vi "Get Calibration Settings.vi"(1 "Channel Settings typedef":T2={"Name"="", "Terminal Information"={"IO Device"=enum."none", "Channel"=0, "Sensor Type"=enum."Voltage"}, "Calibration Information"={"Excitation Voltage"=1.0, "Calibration Factor"=1.0, "Zero Value"=0.0, "Calibration Formula"="(x-x0) / (Ve * CF)", "Units"="V"}}) -> (0 "Calibration Settings ducktype":T1)   [LabVIEW 2021, in "Settings.lvlib"]
uses:
  Acquisition/Channel Settings.ctl
  Acquisition/IO Device.ctl
  Acquisition/Sensor Type.ctl
  Settings.lvlib
  Acquisition/Acquisition.lvlib
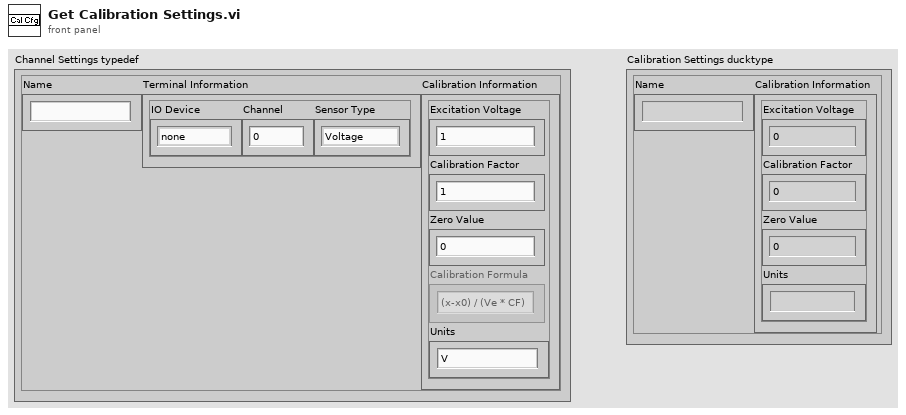
[diagram p1: front panel]
types:
  T1 = cluster{"Name":string, "Calibration Information":cluster{"Excitation Voltage":dbl, "Calibration Factor":dbl, "Zero Value":dbl, "Units":string}}
  T2 = typedef "Acquisition.lvlib/Channel Settings.ctl" = cluster{"Name":string, "Terminal Information":cluster{"IO Device":T3, "Channel":i32, "Sensor Type":T4}, "Calibration Information":cluster{"Excitation Voltage":dbl, "Calibration Factor":dbl, "Zero Value":dbl, "Calibration Formula":string, "Units":string}}
  T3 = typedef "Acquisition.lvlib/IO Device.ctl" = enum16{"none", "9219", "9401"}
  T4 = typedef "Acquisition.lvlib/Sensor Type.ctl" = enum16{"Voltage", "Load", "Pressure", "Encoder"}
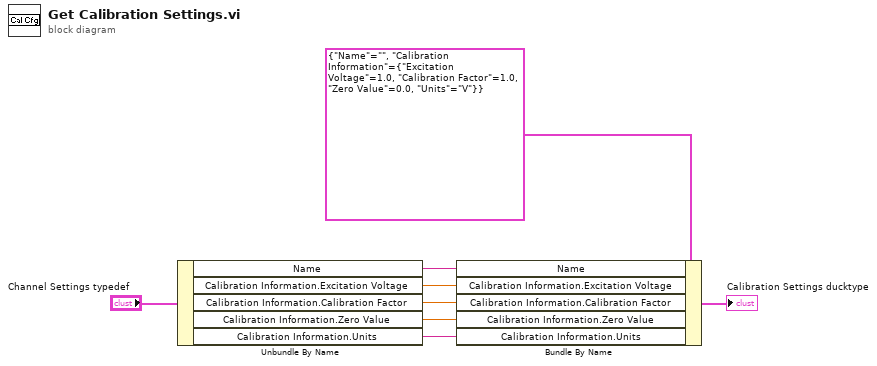
[diagram p0: block diagram]
diagram:
  n1 = Unbundle By Name("Channel Settings typedef") -> ("Name"=w8:string, "Calibration Information.Excitation Voltage"=w6:dbl, "Calibration Information.Calibration Factor"=w5:dbl, "Calibration Information.Zero Value"=w4:dbl, "Calibration Information.Units"=w1:string)
  n2 = Bundle By Name(cluster=T1 {"Name"="", "Calibration Information"={"Excitation Voltage"=1.0, "Calibration Factor"=1.0, "Zero Value"=0.0, "Units"="V"}} ("Channel Settings ducktype"), "Name"=w8, "Calibration Information.Excitation Voltage"=w6, "Calibration Information.Calibration Factor"=w5, "Calibration Information.Zero Value"=w4, "Calibration Information.Units"=w1) -> (→"Calibration Settings ducktype":T1)
